vi "TangoGroup.vi"() -> ()   [LabVIEW 2009]
uses:
  tango_lv9/tango_vi.llb/tango.lvlib
  tango_lv9/tango_vi.llb/avToDoubleScalar.vi
panel:
  out "values":T1(array[cluster])
  out "Waveform Chart":dbl(graph)
  out "Waveform Chart":dbl(graph)
  in  "?":bool=TRUE
  out "attribute name":string
  out "attribute name":string
  out "device name":string
  out "device name":string
  in  "attribute names (will be read on each group member)":string[](array[string])=["short_spectrum_ro", "long_spectrum_ro"]
  out "group id":i32
  in  "group name":string="test_group"
  in  "managed devices":string[](array[string])=["tango/tangotest/*"]
  in  "ignored devices":string[](array[string])
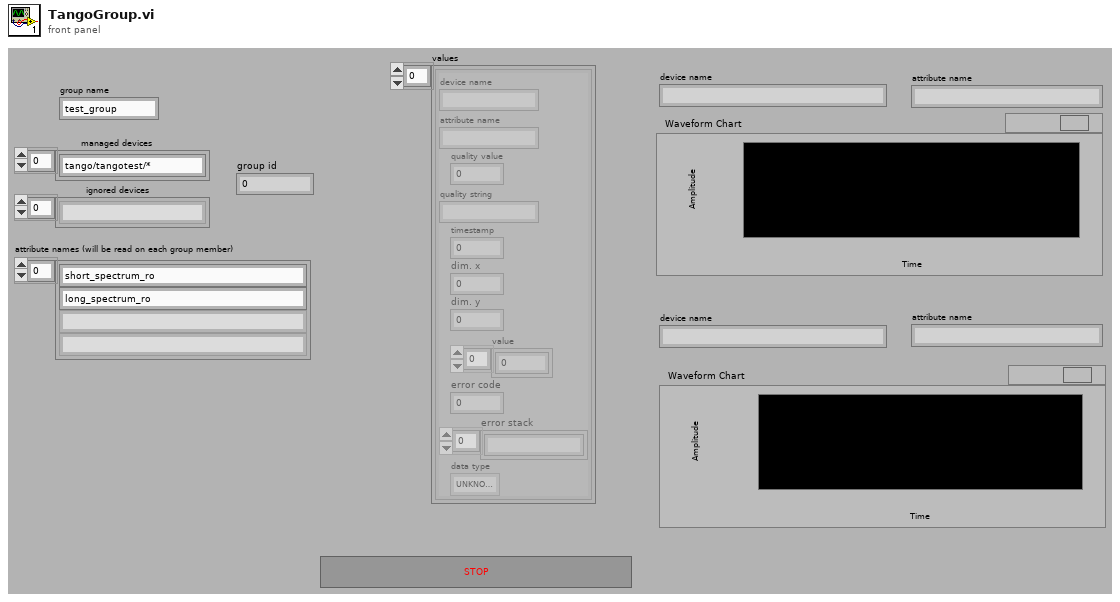
[diagram p1: front panel]
types:
  T1 = cluster{"device name":string, "attribute name":string, "quality value":i16, "quality string":string, "timestamp":dbl, "dim. x":i32, "dim. y":i32, "value":u8[], "error code":i32, "error stack":string[], "data type":enum16{"SCA_STATE", "SCA_STRING", "SPE_STRING", "IMG_STRING", "SCA_BOOLEAN", "SPE_BOOLEAN", "IMG_BOOLEAN", "SCA_UCHAR", "SPE_UCHAR", "IMG_UCHAR", "SCA_SHORT", "SPE_SHORT", "IMG_SHORT", "SCA_USHORT", "SPE_USHORT", "IMG_USHORT", "SCA_LONG", "SPE_LONG", "IMG_LONG", "SCA_ULONG", "SPE_ULONG", "IMG_ULONG", "SCA_FLOAT", "SPE_FLOAT", "IMG_FLOAT", "SCA_DOUBLE", "SPE_DOUBLE", "IMG_DOUBLE", "UNKNOWN_TYPE"}}[]
  T2 = cluster{"device name":string, "attribute name":string, "quality value":i16, "quality string":string, "timestamp":dbl, "dim. x":i32, "dim. y":i32, "value":u8[], "error code":i32, "error stack":string[], "data type":enum16{"SCA_STATE", "SCA_STRING", "SPE_STRING", "IMG_STRING", "SCA_BOOLEAN", "SPE_BOOLEAN", "IMG_BOOLEAN", "SCA_UCHAR", "SPE_UCHAR", "IMG_UCHAR", "SCA_SHORT", "SPE_SHORT", "IMG_SHORT", "SCA_USHORT", "SPE_USHORT", "IMG_USHORT", "SCA_LONG", "SPE_LONG", "IMG_LONG", "SCA_ULONG", "SPE_ULONG", "IMG_ULONG", "SCA_FLOAT", "SPE_FLOAT", "IMG_FLOAT", "SCA_DOUBLE", "SPE_DOUBLE", "IMG_DOUBLE", "UNKNOWN_TYPE"}}
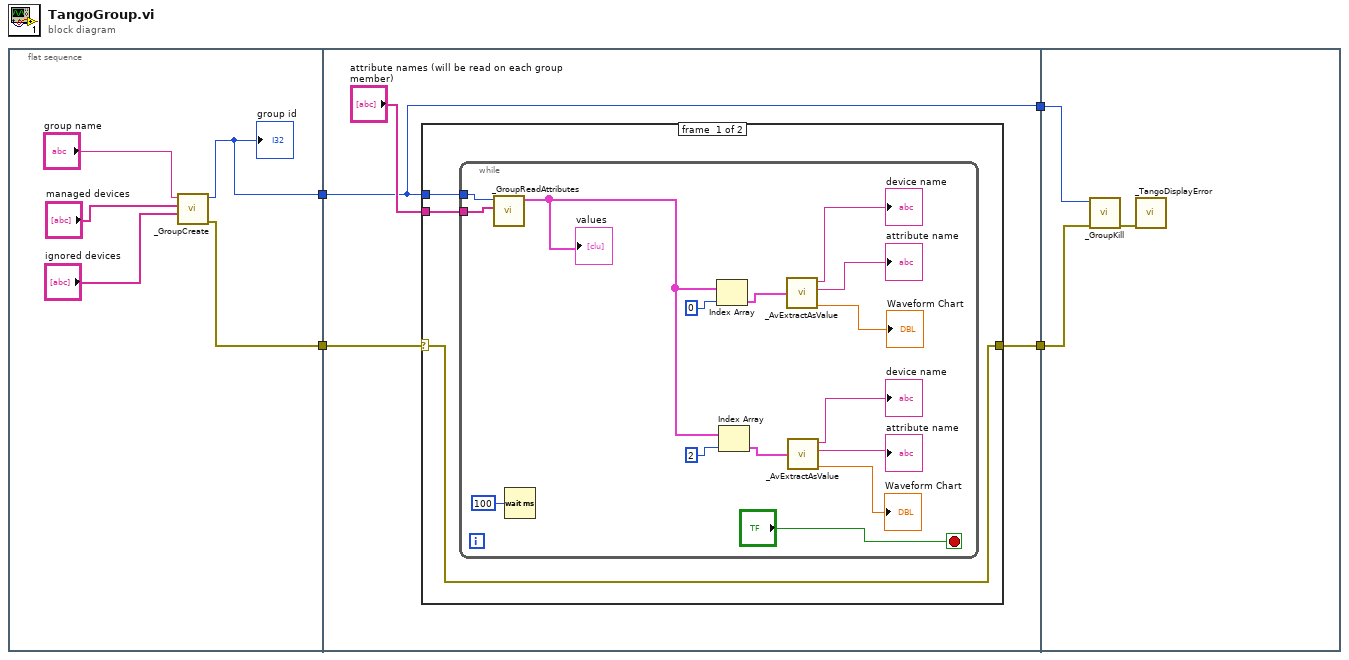
[diagram p0: block diagram]
diagram:
  n1 = flat-sequence {
    tunnel: [w8] -> w4
    tunnel: [w7] -> w2
    tunnel: w4 -> [w12]
    tunnel: [w12] -> w3
    tunnel: w2 -> [w11]
    tunnel: [w10] -> w1
    tunnel: w3 -> [w35]
    tunnel: w1 -> [w34]
    frame #0 {
      n2 = call "_GroupCreate.vi"("ignored devices"="ignored devices", "managed devices"="managed devices", "group name"="group name") -> ("error out"=w7:errorcluster, "group id"=w8:i32)  [unwired: 3 in]
      "group id" <- w8
    }
    frame #1 {
      n3 = case shown="No Error" w11 {
        selector: w11 -> [w14 w32]
        tunnel: "attribute names (will be read on each group member)" -> [w16 _]
        tunnel: w12 -> [w15 _]
        tunnel: [w14 w32] -> w10
        frame #0 {
          n4 = while {
            tunnel: w16 -> [w31]
            tunnel: w15 -> [w30]
            stop <- "?" stop-if-true
            n5 = call "_GroupReadAttributes.vi"("attribute names"=w31, "group id"=w30) -> ("values"=w22:T1)  [unwired: 4 in, 1 out]
            "values" <- w22
            n6 = Wait (ms)(milliseconds to wait=u32 100) -> ()  [unwired: 1 out]
            n7 = Index Array(array=w22, index=0 ("indice")) -> (element=w17:T2)
            n8 = Index Array(array=w22, index=2 ("indice")) -> (element=w18:T2)
            n9 = call-poly "_AvExtractAsValue.vi"("attribute value"=w17) -> ("value"=→"Waveform Chart":dbl, "attribute name"=→"attribute name":string, "device name"=→"device name":string)  [unwired: 2 out]
            n10 = call-poly "_AvExtractAsValue.vi"("attribute value"=w18) -> ("value"=→"Waveform Chart":dbl, "attribute name"=→"attribute name":string, "device name"=→"device name":string)  [unwired: 2 out]
          }
        }
        frame #1 {
        }
      }
    }
    frame #2 {
      n11 = call "_GroupKill.vi"("error in"=w34, "group id"=w35) -> ("error out"=w33:errorcluster)  [unwired: 9 in]
      n12 = call "_TangoDisplayError.vi"("error in"=w33) -> ()  [unwired: 4 in]
    }
  }
